vi "ECHGEI.vi"() -> ()   [LabVIEW 2018]
uses:
  S4GEI/S4GEI.lvclass
  S4GEI/S4GEI.lvclass/S4GEI.ctl
  Channel GUI/Channel.lvclass/Channel.ctl
  Channel GUI/Channel.lvclass
  Camera/Camera.lvclass
panel:
  in  "Tab Control 2":enum32{"Front Panel", "Setup Panel"}(tab)
  in  "Stop Application":bool
  out "Error Message":string
  in  "start exp":bool
  in  "Stop Acquisition":bool
  in  "Abort Acquisition":bool
  in  "Pause acquisition":bool
  in  "exp time":dbl=1.5 min=9.999999747378752e-06
  in  "#frames":u16=1 min=1 max=1000
  in  "#cycles":u32=1 min=1
  in  "Send Message":bool
  in  "Command:":string
  in  "ACS IP":string="200.131.64.25"
  in  "Channel ID":u16=1 min=1
  out "CCD status":T1={"Cycles done"=1, "Frames done"=1, "CCD Status"="", "Exposing"=FALSE, "Last image"="", "temp"=0, "serial n"=0, "texp"=0.0, "used disk"=0, "power"=FALSE, "acs mode"=FALSE} {"Frames done" max=2 scale=0.0..1.0; "Cycles done" max=2 scale=0.0..1.0}
  in  "projid":string="ENG"
  in  "observer":string="Denis"
  in  "object name":string="Test"
  in  "comment":string
  in  "file name suffix":string
  in  "preset modes":T2
  in  "Cooler":bool
  in  "Temp":i32=20 min=-80 max=20
  in  "Set camera configuration":bool
  in  "Readout Rate":u8(ring) items=["1 MHz", "0.1 MHz"]
  in  "Pre-amp gain":u8(ring) items=["Gain 1", "Gain 2", "Error"]
  in  "Vertical Clock Voltagem":u16(ring) items=["Normal", "+1", "+2", "+3", "+4", "Error"]
  in  "Acquisition Mode":u16(ring)=3 items=["Reserved", "Single Scan", "Accumulate", "Kinetic", "Fast Kinetic", "Run till abort", "Reserved", "Reserved", "Reserved", "Time Delayed Integration"]
  in  "Read Mode":u16(ring)=4 items=["Full Vertical Binning", "Multi-Track", "Random-Track", "Single-Track", "Image"]
  in  "Trigger Mode":u16(ring) items=["Internal", "External", "N/A", "N/A", "N/A", "N/A", "External Start", "External Exposure (Bulb)", "N/A", "External FVB EM", "Software", "N/A", "External Charge Shifting"]
  in  "Vertical Shift Speed":u16(ring)=3 items=["0.6", "1.13", "2.2", "4.33", "Error"]
  in  "AD Channel":u16
  in  "Shutter Mode":u8(ring)=2 items=["OPEN"=1, "CLOSED"=2, "Error"=3]
  in  "Shutter Time":u16=50
  in  "Shutter TTL":u16(ring) items=["TTL Low", "TTL High", "Error"]
  in  "Binning":u16=1
  in  "Initial Line":u16=1
  in  "Initial Cloumn":u16=1
  in  "Final Column":u16=1024
  in  "Final Line":u16=1024
  in  "Sub Image":T3(radio)=enum."1024 x 1024"
  # "ECHARPE Graphical Engineering Interface (ECHGEI)"
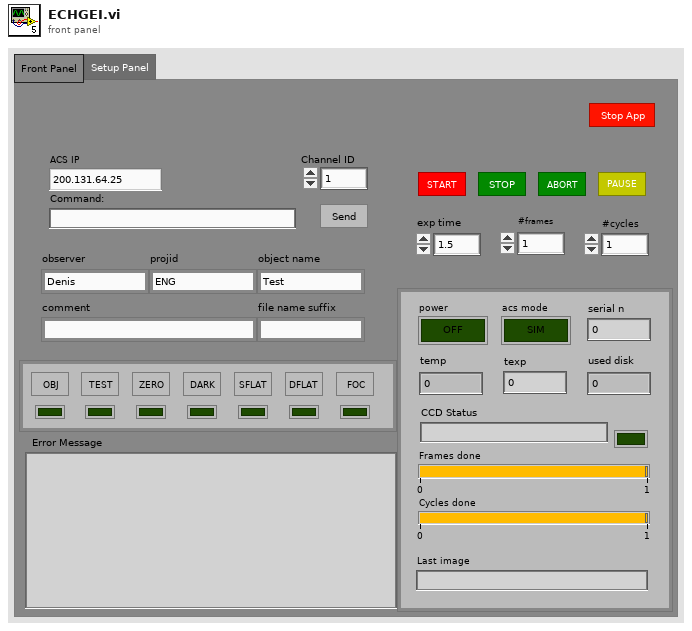
[diagram p1: front panel]
types:
  T1 = cluster{"Cycles done":u16, "Frames done":u16, "CCD Status":string, "Exposing":bool, "Last image":string, "temp":i16, "serial n":u16, "texp":dbl, "used disk":i16, "power":bool, "acs mode":bool}
  T2 = cluster{"OBJECT":bool, "TEST":bool, "ZERO":bool, "DARK":bool, "SFLAT":bool, "DFLAT":bool, "FOCUS":bool, "led object":bool, "led test":bool, "led zero":bool, "led dark":bool, "led sflat":bool, "led dflat":bool, "led foc":bool}
  T3 = enum32{"256 x 256", "512 x 512", "1024 x 1024", "Custom"}
  T4 = cluster{"FWCS IP":string, "ACS IP":string, "Channel ID":u16}
  T5 = cluster{"object":bool, "test":bool, "zero":bool, "dark":bool, "sflat":bool, "dflat":bool, "focus":bool, "object 2":bool, "test 2":bool, "zero 2":bool, "dark 2":bool, "sflat 2":bool, "dflat 2":bool, "foc":bool}
  T6 = enum8{"Enabled", "Disabled", "Disabled and Grayed Out"}
  T7 = cluster{"OBJECT":bool, "TEST":bool, "ZERO":bool, "DARK":bool, "SFLAT":bool, "DFLAT":bool, "FOCUS":bool}
  T8 = cluster{"CYCLES_DONE":u16, "LAST_IMAGE_NAME":string, "USED_DISK_SPACE":u16, "FRAMES_DONE":u16, "CCD_STATUS":string, "CURRENT_TEMPERATURE":i16, "TEMPERATURE_STATUS":string, "FRAME_EXPOSURE_TIME":sgl, "ERROR":bool, "SERIAL_NUMBER":u16, "ACQUIRING":bool, "IMAGE_INDEX":u32, "POWER":bool, "ACS MODE":bool}
  T9 = cluster{"PREAMP":u16, "READOUT_RATE":u16, "VERTICAL_SHIFT_SPEED":u16, "READ_MODE":u16, "VERTICAL_CLOCK_VOLTAGE":u16, "ACQUISITION_MODE":u16, "AD_CHANNEL":u16, "SHUTTER_TTL":u16, "SHUTTER_OPENING_TIME":u16, "SHUTTER_CLOSING_TIME":u16, "SHUTTER_MODE":u16, "TRIGGER_MODE":u16, "VBIN":u16, "INITIAL_LINE":u16, "INITIAL_COLUMN":u16, "FINAL_LINE":u16, "FINAL_COLUMN":u16, "HBIN":u16}
  T10 = cluster{"EXPTIME":dbl, "#FRAMES":u32, "#CYCLES":u32, "suffix":string, "TEMP":i32, "COOLER_POWER_STATUS":u16}
  T11 = cluster{"Acquire":bool, "Stop Acquisition":bool, "Abort Acquisition":bool, "Pause acquisition":bool}
  T12 = cluster{"OBJECT":string, "OBSERVER":string, "CTRLINTE":string, "PROJID":string, "SYNCMODE":string, "INSTMODE":string, "FILTER":string, "OBSTYPE":string, "GUIVRSN":string, "COMMENT":string, "broker":string, "timestamp":string, "CHANNEL 1":bool, "CHANNEL 2":bool, "CHANNEL 3":bool, "CHANNEL 4":bool, "TCSMODE":bool}
  T13 = cluster{"Cycles done":u16, "Frames done":u16, "CCD Status":string, "Exposing":bool, "Last image":string, "temp":i16, "serial n":u16, "texp":dbl, "used disk":i16, "Power":bool, "ACS mode":bool}
  T14 = cluster{"object":bool, "test":bool, "zero":bool, "dark":bool, "sflat":bool, "dflat":bool, "focus":bool, "led object":bool, "led test":bool, "led zero":bool, "led dark":bool, "led sflat":bool, "led dflat":bool, "led foc":bool}
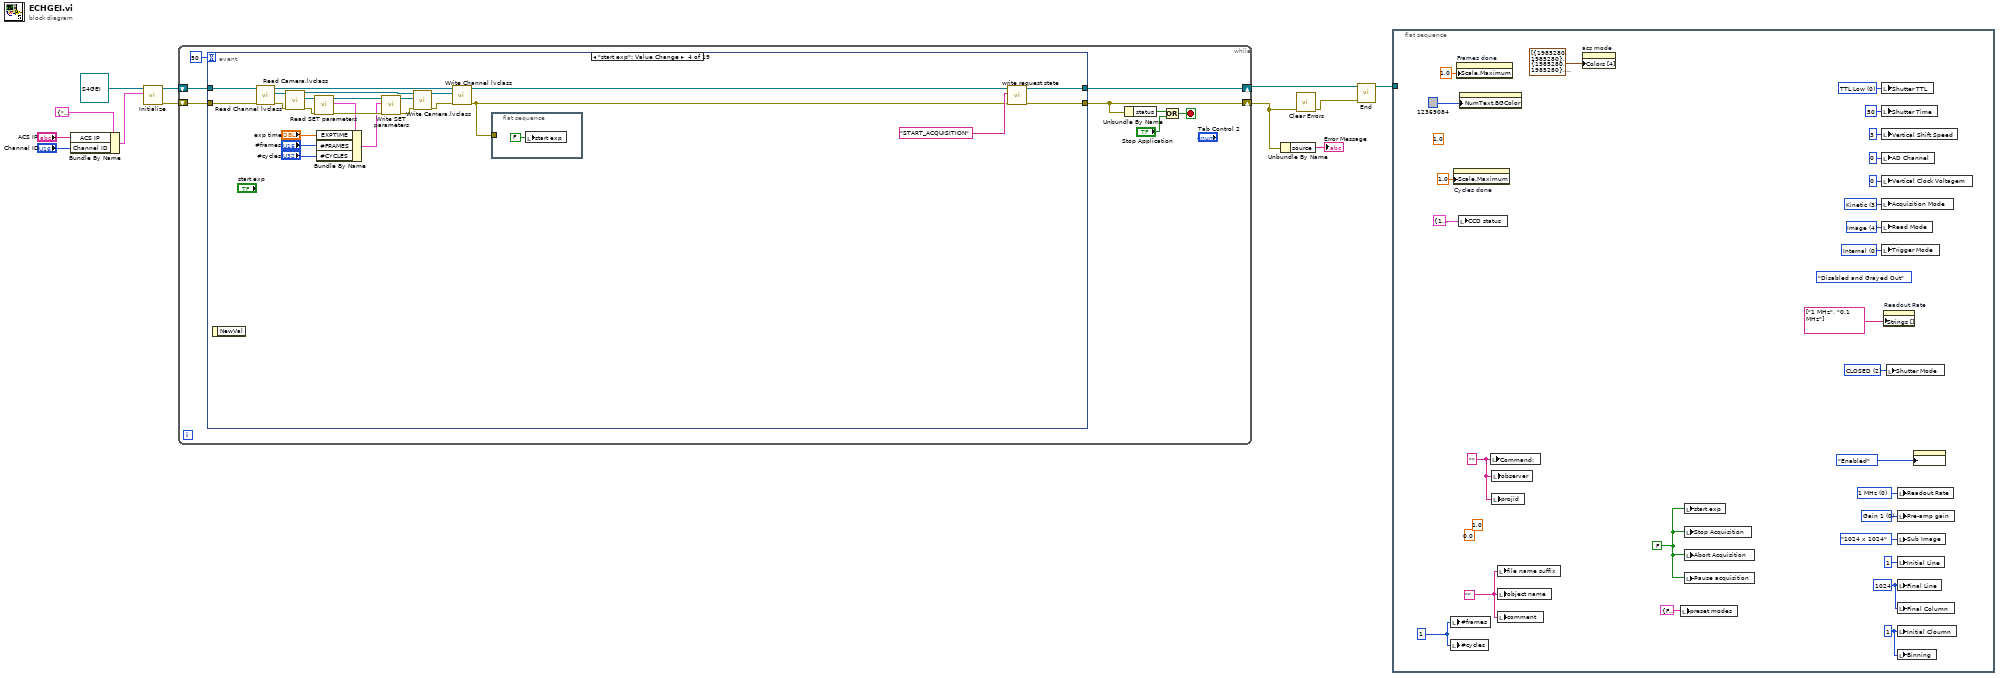
[diagram p0: block diagram]
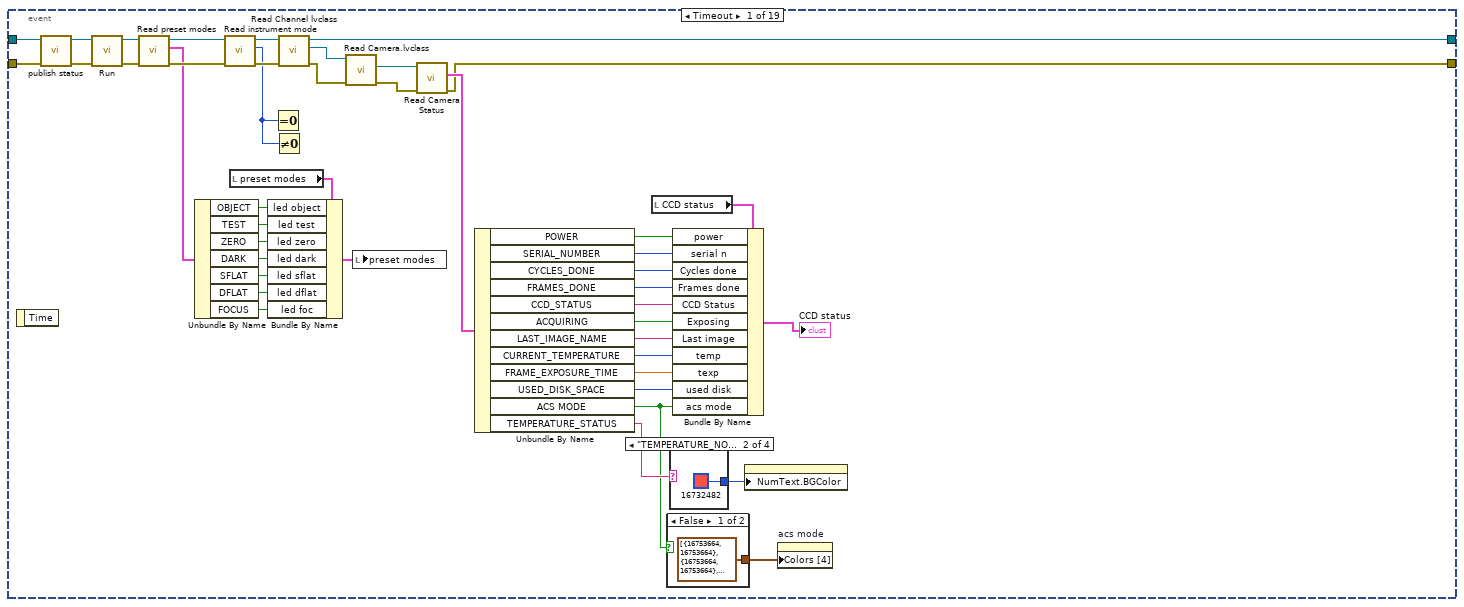
[diagram p2: hidden frame]
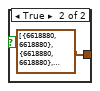
[diagram p3: hidden frame]
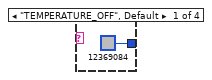
[diagram p4: hidden frame]
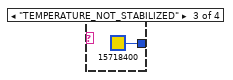
[diagram p5: hidden frame]
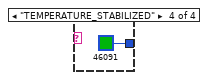
[diagram p6: hidden frame]
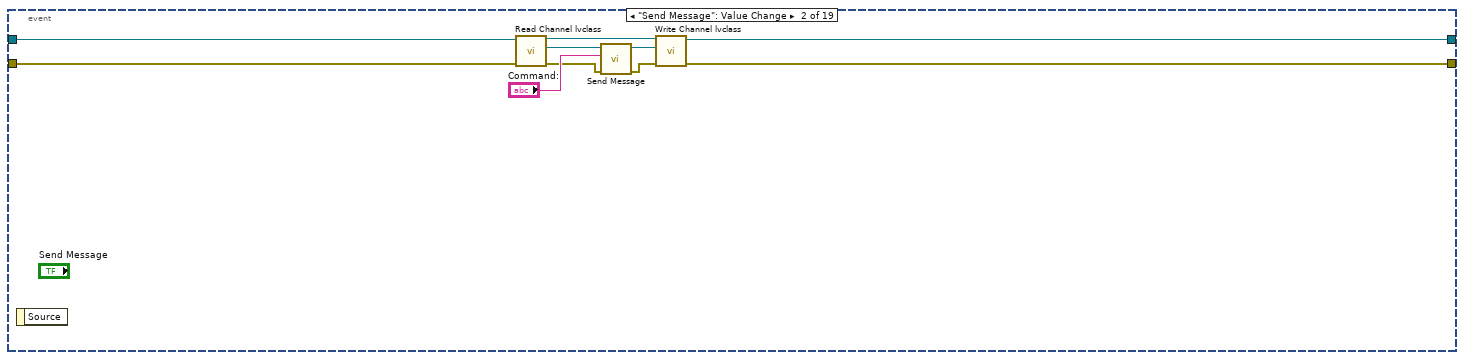
[diagram p7: hidden frame]
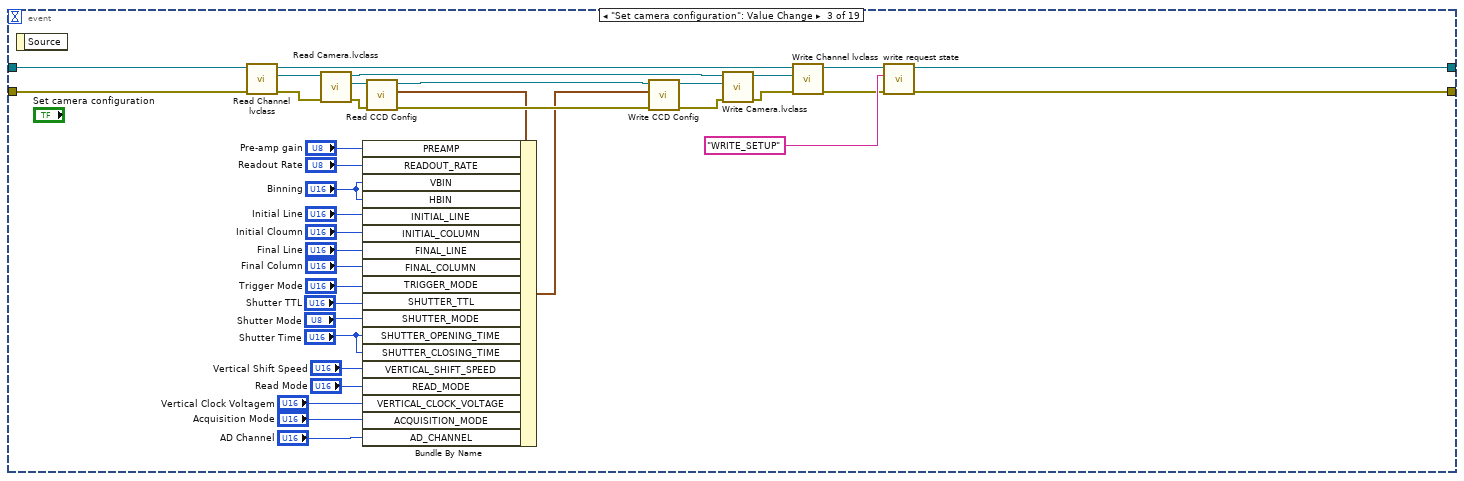
[diagram p8: hidden frame]
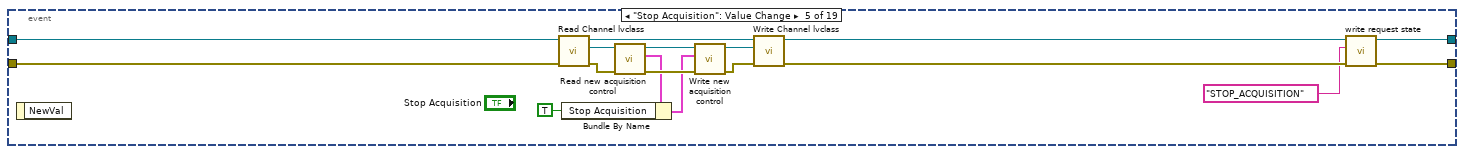
[diagram p9: hidden frame]
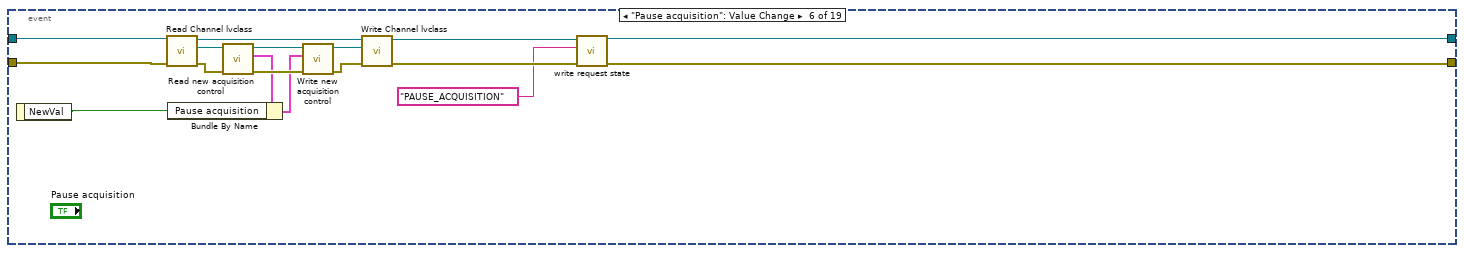
[diagram p10: hidden frame]
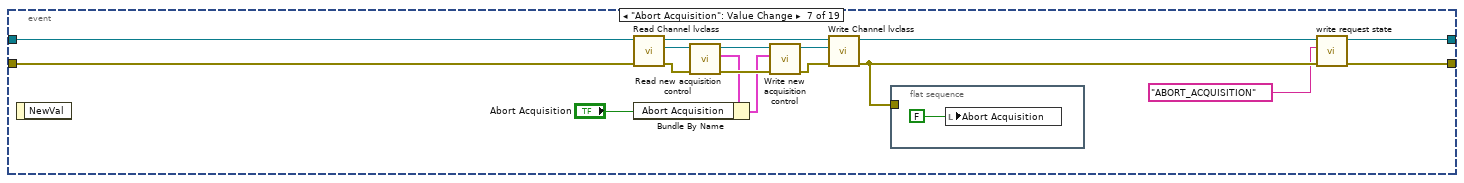
[diagram p11: hidden frame]
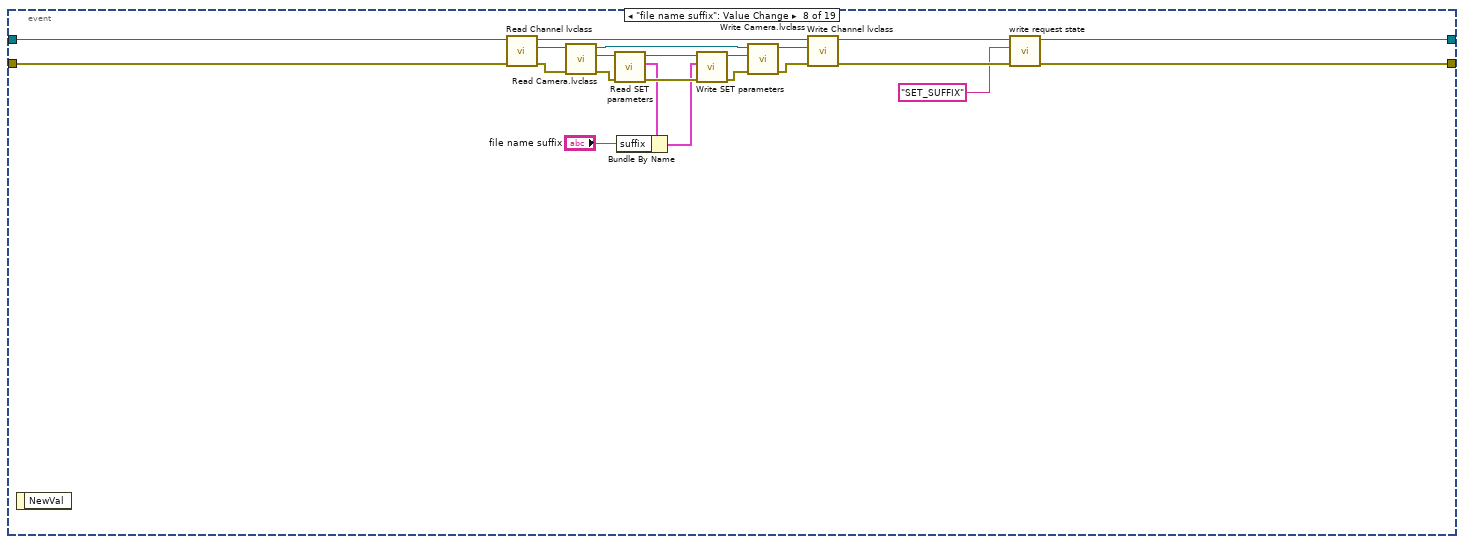
[diagram p12: hidden frame]
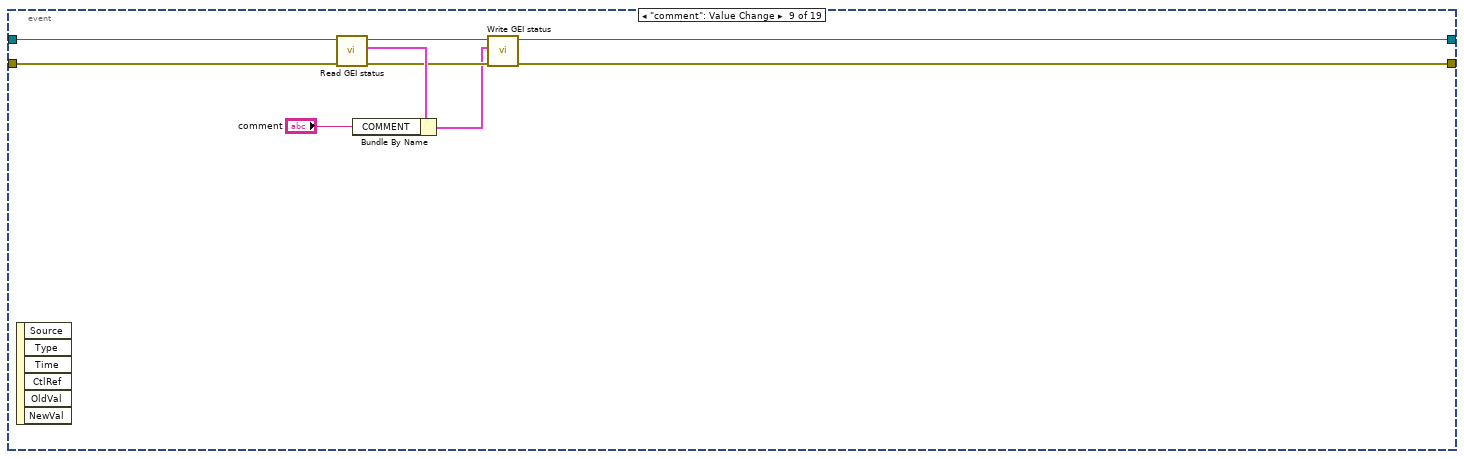
[diagram p13: hidden frame]
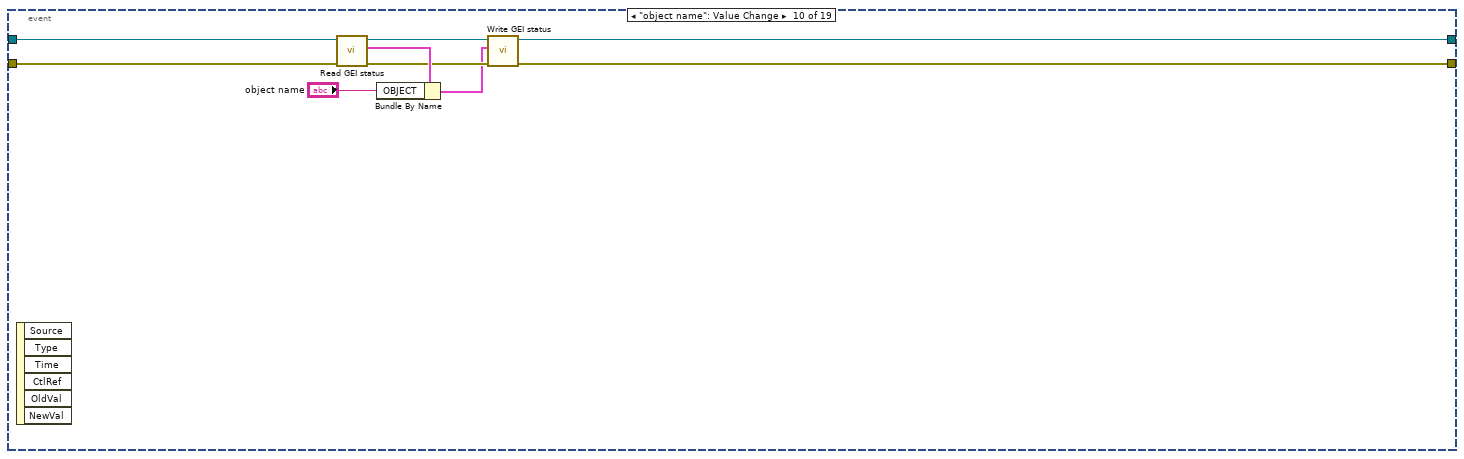
[diagram p14: hidden frame]
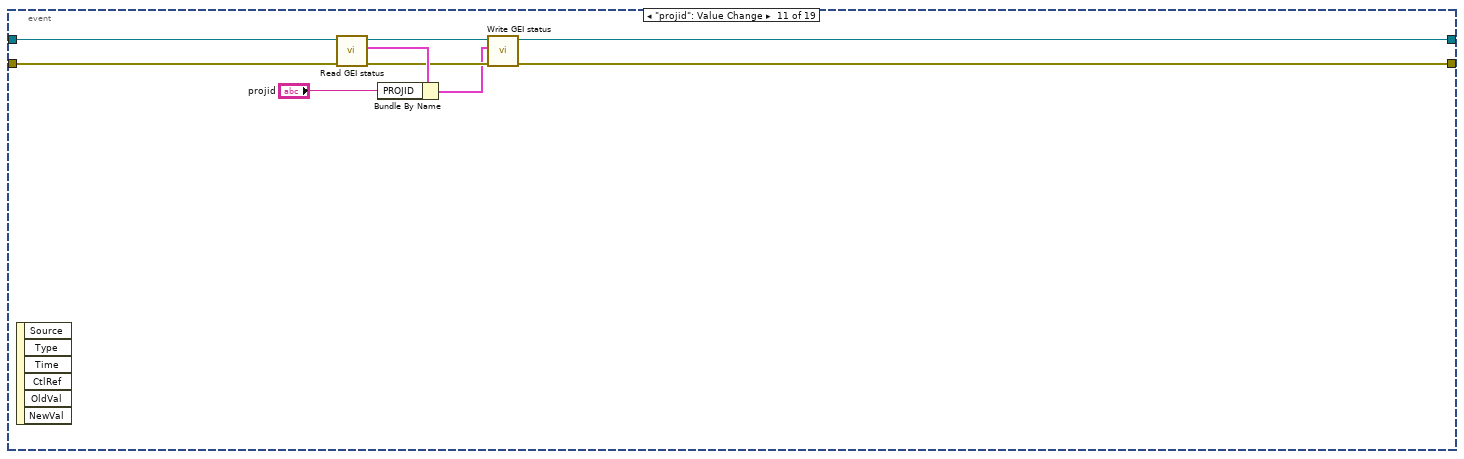
[diagram p15: hidden frame]
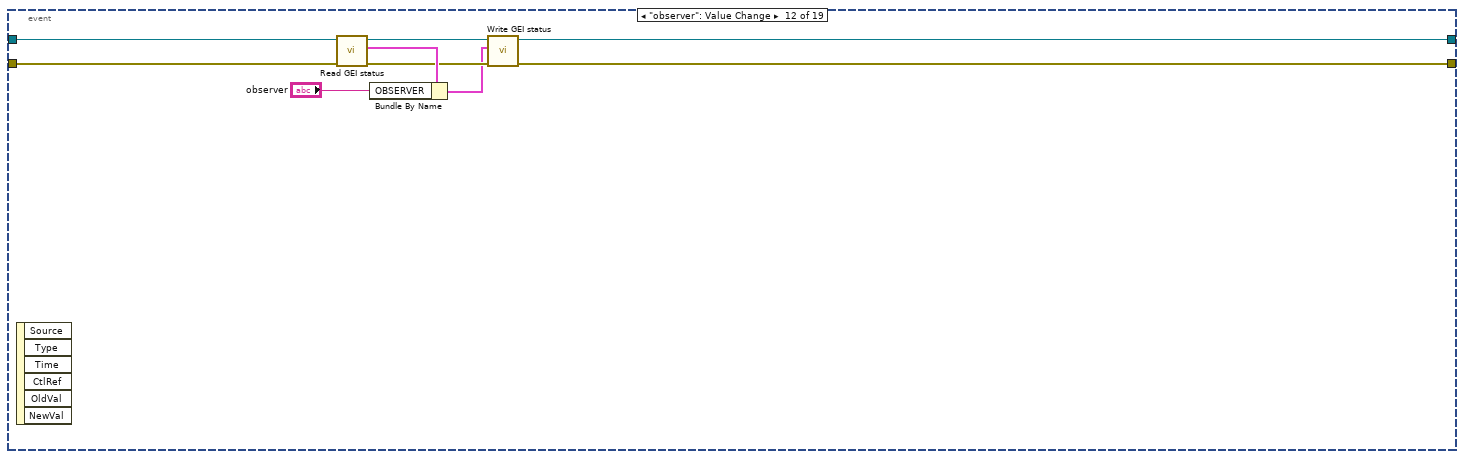
[diagram p16: hidden frame]
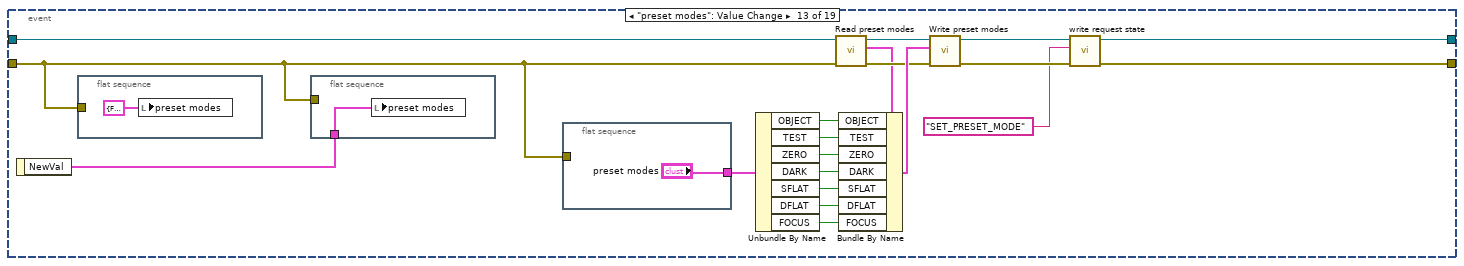
[diagram p17: hidden frame]
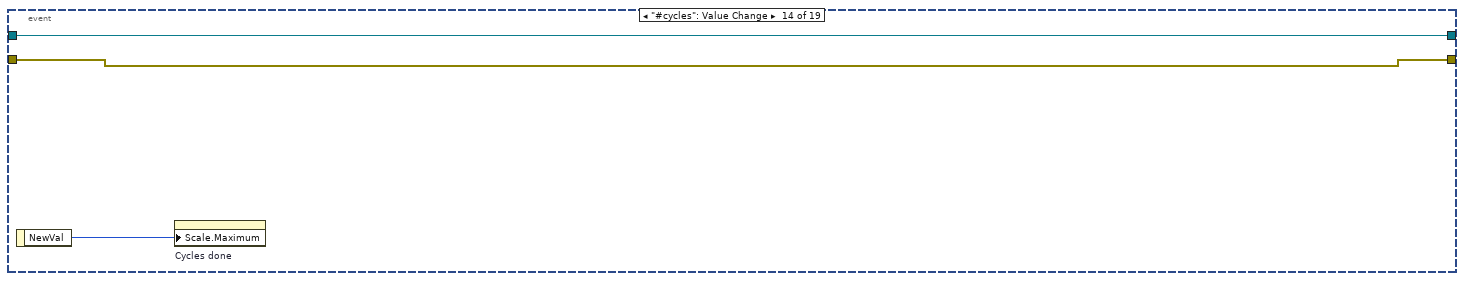
[diagram p18: hidden frame]
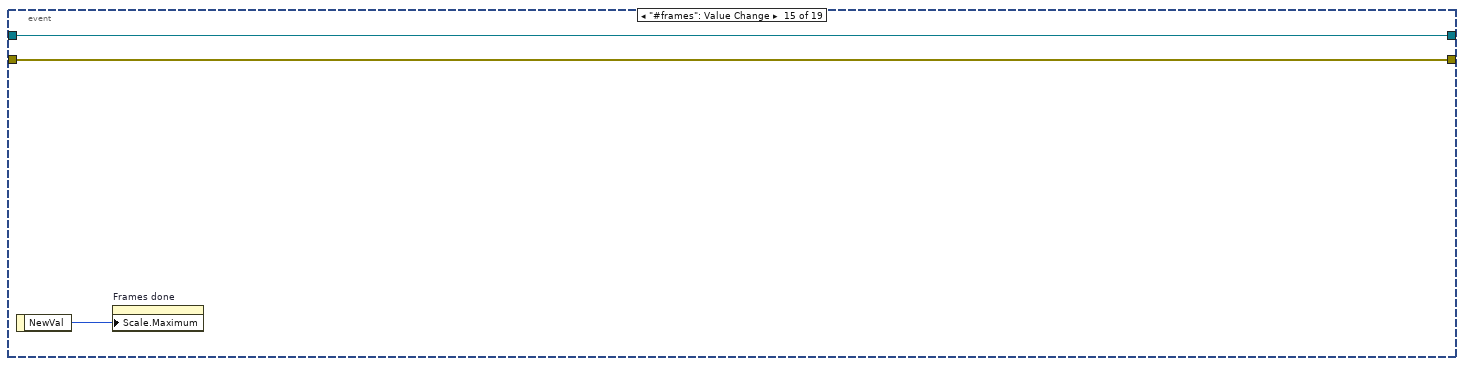
[diagram p19: hidden frame]
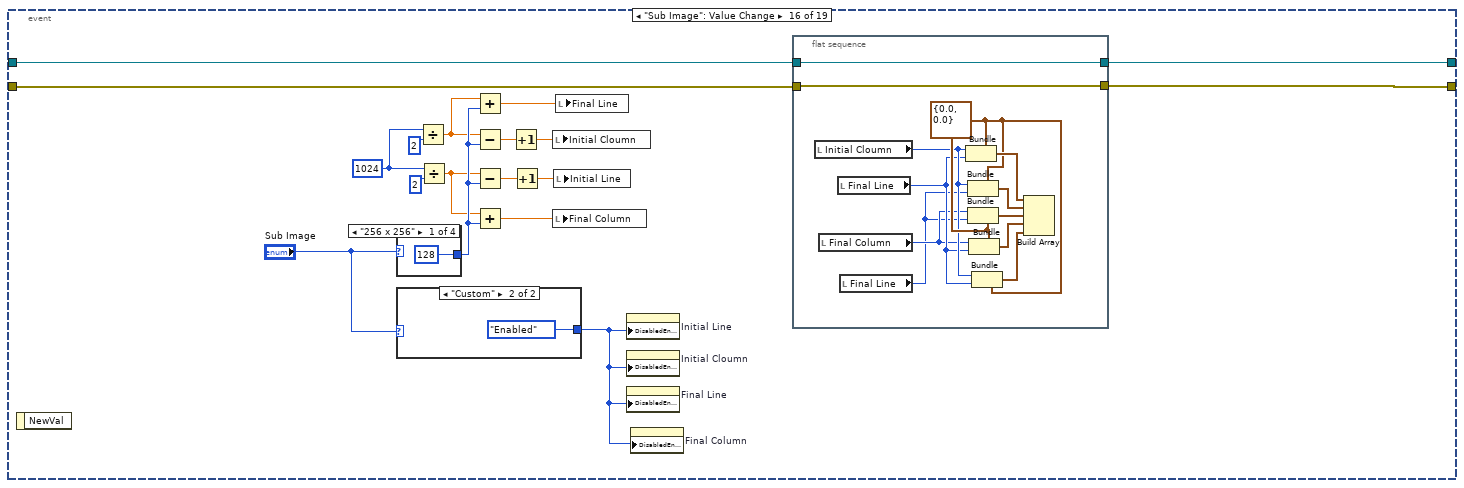
[diagram p20: hidden frame]
diagram:
  n1 = Bundle By Name(cluster=T4 {"FWCS IP"="200.131.64.49", "ACS IP"="200.131.64.25", "Channel ID"=1} ("Communication variables"), "ACS IP"="ACS IP", "Channel ID"="Channel ID") -> (w6:T4)
  n2 = call "Initialize.vi"("Communication variables"=w6, "SPARC4_GUI in"=refnum<class "S4GEI.lvclass"> refnum ("SPARC4_GUI.lvclass")) -> ("error out"=w2:errorcluster, "SPARC4_GUI out"=w1:refnum<class "S4GEI.lvclass">)  [unwired: 8 in]
  n3 = while {
    shift-right: [w13] -> w9
    shift-left: w2 -> [w15]
    shift-right: [w14] -> w11
    shift-left: w1 -> [w16]
    stop <- w19 stop-if-true
    n4 = event shown="[3] \"start exp\": Value Change" {
      selector: _ -> [_ _ _ _ _ _ _ _ _ _ _ _ _ _ _ _ _ _ _]
      dyn-events: _ -> [_ _ _ _ _ _ _ _ _ _ _ _ _ _ _ _ _ _ _]
      timeout: 50 -> [_ _ _ _ _ _ _ _ _ _ _ _ _ _ _ _ _ _ _]
      tunnel: w15 -> [w61 w78 w116 w139 w157 w166 w183 w215 w222 w231 w240 w249 w262 w277 w280 w298 w321 w339 w361]
      tunnel: [w40 w71 w82 w124 w147 w162 w178 w196 w223 w232 w241 w250 w269 w277 w280 w296 w321 w325 w349] -> w13
      tunnel: w16 -> [w62 w79 w117 w140 w158 w167 w184 w214 w224 w233 w242 w251 w261 w278 w281 w299 w320 w340 w362]
      tunnel: [w44 w72 w81 w125 w148 w161 w179 w197 w225 w234 w243 w252 w268 w278 w281 w297 w320 w326 w350] -> w14
      event Timeout {
        n5 = event-data() -> ()  [unwired: 1 in, 1 out]
        n6 = call "publish status.vi"("error in (no error)"=w61, "S4GEI in"=w62) -> ("error out"=w60:errorcluster, "S4GEI out"=w59:refnum<class "S4GEI.lvclass">)  [unwired: 8 in]
        n7 = call "Run.vi"("error in (no error)"=w60, "SPARC4_GUI in"=w59) -> ("error out"=w36:errorcluster, "SPARC4_GUI out"=w39:refnum<class "S4GEI.lvclass">)  [unwired: 8 in]
        n8 = call-dynamic "Read preset modes.vi"("error in (no error)"=w36, "S4GEI in"=w39) -> ("error out"=w37:errorcluster, "preset modes"=w33:T7, "S4GEI out"=w38:refnum<class "S4GEI.lvclass">)  [unwired: 7 in]
        n9 = Unbundle By Name(w33) -> ("OBJECT"=w26:bool, "TEST"=w27:bool, "ZERO"=w28:bool, "DARK"=w29:bool, "SFLAT"=w30:bool, "DFLAT"=w31:bool, "FOCUS"=w32:bool)
        n10 = call-dynamic "Read instrument mode.vi"("error in (no error)"=w37, "S4GEI in"=w38) -> ("error out"=w42:errorcluster, "instrument mode"=w41:u16, "S4GEI out"=w43:refnum<class "S4GEI.lvclass">)  [unwired: 7 in]
        n11 = local read "preset modes"() -> (w35:T2)
        n12 = Bundle By Name(cluster=w35, "led object"=w26, "led test"=w27, "led zero"=w28, "led dark"=w29, "led sflat"=w30, "led dflat"=w31, "led foc"=w32) -> (w34:T2)
        n13 = Equal To 0?(x=w41) -> ()  [unwired: 1 out]
        n14 = Not Equal To 0?(x=w41) -> ()  [unwired: 1 out]
        n15 = call "Read Channel lvclass.vi"("error in (no error)"=w42, "SPARC4_GUI in"=w43) -> ("error out"=w56:errorcluster, "Channel.lvclass"=w58:refnum<class "Channel.lvclass">, "SPARC4_GUI out"=w44:refnum<class "S4GEI.lvclass">)  [unwired: 7 in]
        n16 = call-dynamic "Read Camera.lvclass.vi"("error in (no error)"=w56, "Channel in"=w58) -> ("error out"=w55:errorcluster, "Camera.lvclass"=w57:refnum<class "Camera.lvclass">)  [unwired: 7 in, 1 out]
        n17 = local write "preset modes"(w34) -> ()
        n18 = call-dynamic "Read Camera Status.vi"("error in (no error)"=w55, "Camera in"=w57) -> ("error out"=w40:errorcluster, "Camera Status"=w63:T8)  [unwired: 7 in, 1 out]
        n19 = Unbundle By Name(w63) -> ("POWER"=w24:bool, "SERIAL_NUMBER"=w25:u16, "CYCLES_DONE"=w52:u16, "FRAMES_DONE"=w51:u16, "CCD_STATUS"=w50:string, "ACQUIRING"=w49:bool, "LAST_IMAGE_NAME"=w48:string, "CURRENT_TEMPERATURE"=w47:i16, "FRAME_EXPOSURE_TIME"=w46:sgl, "USED_DISK_SPACE"=w45:u16, "ACS MODE"=w21:bool, "TEMPERATURE_STATUS"=w23:string)
        n20 = local read "CCD status"() -> (w54:T1)
        n21 = case shown="False" w21 {
          tunnel: [cluster{u32, u32}[] [{16753664, 16753664}, {16753664, 16753664}, {16753664, 16753664}] ("Colors [4]") cluster{u32, u32}[] [{6618880, 6618880}, {6618880, 6618880}, {6618880, 6618880}] ("Colors [4]")] -> w22
          frame False {
          }
          frame True {
          }
        }
        n22 = case shown="\"TEMPERATURE_NOT_REACHED\"" w23 {
          tunnel: [u32 12369084 u32 16732482 u32 15718400 u32 46091] -> w64
          frame "TEMPERATURE_OFF", Default {
          }
          frame "TEMPERATURE_NOT_REACHED" {
          }
          frame "TEMPERATURE_NOT_STABILIZED" {
          }
          frame "TEMPERATURE_STABILIZED" {
          }
        }
        n23 = Bundle By Name(cluster=w54, "power"=w24, "serial n"=w25, "Cycles done"=w52, "Frames done"=w51, "CCD Status"=w50, "Exposing"=w49, "Last image"=w48, "temp"=w47, "texp"=w46, "used disk"=w45, "acs mode"=w21) -> (→"CCD status":T1)
        n24 = property on="temp" class="DigNum (strict)"("NumText.BGColor"=w64) -> ()  [unwired: 2 in, 2 out]
        n25 = property on="acs mode" class="Bool (strict)"("Colors [4]"=w22) -> ()  [unwired: 2 in, 2 out]
      }
      event "Send Message": Value Change {
        n26 = event-data() -> ()  [unwired: 1 in, 1 out]
        n27 = call "Read Channel lvclass.vi"("error in (no error)"=w78, "SPARC4_GUI in"=w79) -> ("error out"=w74:errorcluster, "Channel.lvclass"=w77:refnum<class "Channel.lvclass">, "SPARC4_GUI out"=w73:refnum<class "S4GEI.lvclass">)  [unwired: 7 in]
        n28 = call "Send Message.vi"("error in (no error)"=w74, "Message"="Command:", "Channel GUI in"=w77) -> ("error out"=w75:errorcluster, "Channel GUI out"=w76:refnum<class "Channel.lvclass">)  [unwired: 7 in]
        n29 = call "Write Channel lvclass.vi"("error in (no error)"=w75, "Channel.lvclass"=w76, "SPARC4_GUI in"=w73) -> ("error out"=w71:errorcluster, "SPARC4_GUI out"=w72:refnum<class "S4GEI.lvclass">)  [unwired: 7 in]
      }
      event "Set camera configuration": Value Change {
        n30 = event-data() -> ()  [unwired: 1 in, 1 out]
        n31 = call "Read Channel lvclass.vi"("error in (no error)"=w116, "SPARC4_GUI in"=w117) -> ("error out"=w115:errorcluster, "Channel.lvclass"=w87:refnum<class "Channel.lvclass">, "SPARC4_GUI out"=w114:refnum<class "S4GEI.lvclass">)  [unwired: 7 in]
        n32 = call-dynamic "Read Camera.lvclass.vi"("error in (no error)"=w115, "Channel in"=w87) -> ("error out"=w113:errorcluster, "Camera.lvclass"=w112:refnum<class "Camera.lvclass">, "Channel out"=w86:refnum<class "Channel.lvclass">)  [unwired: 7 in]
        n33 = call-dynamic "Read CCD Config.vi"("error in (no error)"=w113, "Camera in"=w112) -> ("error out"=w111:errorcluster, "CCD Config"=w89:T9, "Camera out"=w94:refnum<class "Camera.lvclass">)  [unwired: 7 in]
        n34 = Bundle By Name(cluster=w89, "PREAMP"="Pre-amp gain", "READOUT_RATE"="Readout Rate", "VBIN"="Binning", "HBIN"="Binning", "INITIAL_LINE"="Initial Line", "INITIAL_COLUMN"="Initial Cloumn", "FINAL_LINE"="Final Line", "FINAL_COLUMN"="Final Column", "TRIGGER_MODE"="Trigger Mode", "SHUTTER_TTL"="Shutter TTL", "SHUTTER_MODE"="Shutter Mode", "SHUTTER_OPENING_TIME"="Shutter Time", "SHUTTER_CLOSING_TIME"="Shutter Time", "VERTICAL_SHIFT_SPEED"="Vertical Shift Speed", "READ_MODE"="Read Mode", "VERTICAL_CLOCK_VOLTAGE"="Vertical Clock Voltagem", "ACQUISITION_MODE"="Acquisition Mode", "AD_CHANNEL"="AD Channel") -> (w88:T9)
        n35 = call-dynamic "Write CCD Config.vi"("error in (no error)"=w111, "CCD Config"=w88, "Camera in"=w94) -> ("error out"=w92:errorcluster, "Camera out"=w93:refnum<class "Camera.lvclass">)  [unwired: 7 in]
        n36 = call-dynamic "Write Camera.lvclass.vi"("error in (no error)"=w92, "Camera.lvclass"=w93, "Channel in"=w86) -> ("error out"=w91:errorcluster, "Channel out"=w90:refnum<class "Channel.lvclass">)  [unwired: 7 in]
        n37 = call "Write Channel lvclass.vi"("error in (no error)"=w91, "Channel.lvclass"=w90, "SPARC4_GUI in"=w114) -> ("error out"=w84:errorcluster, "SPARC4_GUI out"=w83:refnum<class "S4GEI.lvclass">)  [unwired: 7 in]
        n38 = call "write request state.vi"("error in (no error)"=w84, "State"="WRITE_SETUP", "S4GEI in"=w83) -> ("error out"=w82:errorcluster, "S4GEI out"=w81:refnum<class "S4GEI.lvclass">)  [unwired: 7 in]
      }
      event "start exp": Value Change {
        n39 = event-data() -> ()  [unwired: 1 in, 1 out]
        n40 = call "Read Channel lvclass.vi"("error in (no error)"=w139, "SPARC4_GUI in"=w140) -> ("error out"=w138:errorcluster, "Channel.lvclass"=w127:refnum<class "Channel.lvclass">, "SPARC4_GUI out"=w141:refnum<class "S4GEI.lvclass">)  [unwired: 7 in]
        n41 = call-dynamic "Read Camera.lvclass.vi"("error in (no error)"=w138, "Channel in"=w127) -> ("error out"=w134:errorcluster, "Camera.lvclass"=w135:refnum<class "Camera.lvclass">, "Channel out"=w126:refnum<class "Channel.lvclass">)  [unwired: 7 in]
        n42 = call-dynamic "Read SET parameters.vi"("error in (no error)"=w134, "Camera in"=w135) -> ("error out"=w132:errorcluster, "SET parameters"=w129:T10, "Camera out"=w133:refnum<class "Camera.lvclass">)  [unwired: 7 in]
        n43 = Bundle By Name(cluster=w129, "EXPTIME"="exp time", "#FRAMES"="#frames", "#CYCLES"="#cycles") -> (w128:T10)
        n44 = call-dynamic "Write SET parameters.vi"("error in (no error)"=w132, "SET parameters"=w128, "Camera in"=w133) -> ("error out"=w130:errorcluster, "Camera out"=w131:refnum<class "Camera.lvclass">)  [unwired: 7 in]
        n45 = call-dynamic "Write Camera.lvclass.vi"("error in (no error)"=w130, "Camera.lvclass"=w131, "Channel in"=w126) -> ("error out"=w137:errorcluster, "Channel out"=w136:refnum<class "Channel.lvclass">)  [unwired: 7 in]
        n46 = call "Write Channel lvclass.vi"("error in (no error)"=w137, "Channel.lvclass"=w136, "SPARC4_GUI in"=w141) -> ("error out"=w121:errorcluster, "SPARC4_GUI out"=w122:refnum<class "S4GEI.lvclass">)  [unwired: 7 in]
        n47 = flat-sequence {
          tunnel: w121 -> [_]
          frame #0 {
            n48 = local write "start exp"(FALSE ("start exp")) -> ()
          }
        }
        n49 = call "write request state.vi"("error in (no error)"=w121, "State"="START_ACQUISITION", "S4GEI in"=w122) -> ("error out"=w124:errorcluster, "S4GEI out"=w125:refnum<class "S4GEI.lvclass">)  [unwired: 7 in]
      }
      event "Stop Acquisition": Value Change {
        n50 = event-data() -> ()  [unwired: 1 in, 1 out]
        n51 = call "Read Channel lvclass.vi"("error in (no error)"=w157, "SPARC4_GUI in"=w158) -> ("error out"=w153:errorcluster, "Channel.lvclass"=w156:refnum<class "Channel.lvclass">, "SPARC4_GUI out"=w159:refnum<class "S4GEI.lvclass">)  [unwired: 7 in]
        n52 = call "Read new acquisition control.vi"("error in (no error)"=w153, "Channel in"=w156) -> ("error out"=w152:errorcluster, "new acquisition control"=w150:T11, "Channel out"=w155:refnum<class "Channel.lvclass">)  [unwired: 7 in]
        n53 = Bundle By Name(cluster=w150, "Stop Acquisition"=TRUE) -> (w149:T11)
        n54 = call "Write new acquisition control.vi"("error in (no error)"=w152, "new acquisition control"=w149, "Channel in"=w155) -> ("error out"=w151:errorcluster, "Channel out"=w154:refnum<class "Channel.lvclass">)  [unwired: 7 in]
        n55 = call "Write Channel lvclass.vi"("error in (no error)"=w151, "Channel.lvclass"=w154, "SPARC4_GUI in"=w159) -> ("error out"=w146:errorcluster, "SPARC4_GUI out"=w145:refnum<class "S4GEI.lvclass">)  [unwired: 7 in]
        n56 = call "write request state.vi"("error in (no error)"=w146, "State"="STOP_ACQUISITION", "S4GEI in"=w145) -> ("error out"=w147:errorcluster, "S4GEI out"=w148:refnum<class "S4GEI.lvclass">)  [unwired: 7 in]
      }
      event "Pause acquisition": Value Change {
        n57 = event-data() -> ("NewVal"=w165:bool)  [unwired: 1 in]
        n58 = call "Read Channel lvclass.vi"("error in (no error)"=w166, "SPARC4_GUI in"=w167) -> ("error out"=w172:errorcluster, "Channel.lvclass"=w175:refnum<class "Channel.lvclass">, "SPARC4_GUI out"=w176:refnum<class "S4GEI.lvclass">)  [unwired: 7 in]
        n59 = call "Read new acquisition control.vi"("error in (no error)"=w172, "Channel in"=w175) -> ("error out"=w171:errorcluster, "new acquisition control"=w169:T11, "Channel out"=w174:refnum<class "Channel.lvclass">)  [unwired: 7 in]
        n60 = Bundle By Name(cluster=w169, "Pause acquisition"=w165) -> (w168:T11)
        n61 = call "Write new acquisition control.vi"("error in (no error)"=w171, "new acquisition control"=w168, "Channel in"=w174) -> ("error out"=w170:errorcluster, "Channel out"=w173:refnum<class "Channel.lvclass">)  [unwired: 7 in]
        n62 = call "Write Channel lvclass.vi"("error in (no error)"=w170, "Channel.lvclass"=w173, "SPARC4_GUI in"=w176) -> ("error out"=w164:errorcluster, "SPARC4_GUI out"=w163:refnum<class "S4GEI.lvclass">)  [unwired: 7 in]
        n63 = call "write request state.vi"("error in (no error)"=w164, "State"="PAUSE_ACQUISITION", "S4GEI in"=w163) -> ("error out"=w162:errorcluster, "S4GEI out"=w161:refnum<class "S4GEI.lvclass">)  [unwired: 7 in]
      }
      event "Abort Acquisition": Value Change {
        n64 = event-data() -> ()  [unwired: 1 in, 1 out]
        n65 = call "Read Channel lvclass.vi"("error in (no error)"=w183, "SPARC4_GUI in"=w184) -> ("error out"=w189:errorcluster, "Channel.lvclass"=w192:refnum<class "Channel.lvclass">, "SPARC4_GUI out"=w193:refnum<class "S4GEI.lvclass">)  [unwired: 7 in]
        n66 = call "Read new acquisition control.vi"("error in (no error)"=w189, "Channel in"=w192) -> ("error out"=w188:errorcluster, "new acquisition control"=w186:T11, "Channel out"=w191:refnum<class "Channel.lvclass">)  [unwired: 7 in]
        n67 = Bundle By Name(cluster=w186, "Abort Acquisition"="Abort Acquisition") -> (w185:T11)
        n68 = call "Write new acquisition control.vi"("error in (no error)"=w188, "new acquisition control"=w185, "Channel in"=w191) -> ("error out"=w187:errorcluster, "Channel out"=w190:refnum<class "Channel.lvclass">)  [unwired: 7 in]
        n69 = call "Write Channel lvclass.vi"("error in (no error)"=w187, "Channel.lvclass"=w190, "SPARC4_GUI in"=w193) -> ("error out"=w180:errorcluster, "SPARC4_GUI out"=w181:refnum<class "S4GEI.lvclass">)  [unwired: 7 in]
        n70 = flat-sequence {
          tunnel: w180 -> [_]
          frame #0 {
            n71 = local write "Abort Acquisition"(FALSE ("Abort Acquisition")) -> ()
          }
        }
        n72 = call "write request state.vi"("error in (no error)"=w180, "State"="ABORT_ACQUISITION", "S4GEI in"=w181) -> ("error out"=w178:errorcluster, "S4GEI out"=w179:refnum<class "S4GEI.lvclass">)  [unwired: 7 in]
      }
      event "file name suffix": Value Change {
        n73 = event-data() -> ()  [unwired: 1 in, 1 out]
        n74 = call "Read Channel lvclass.vi"("error in (no error)"=w215, "SPARC4_GUI in"=w214) -> ("error out"=w213:errorcluster, "Channel.lvclass"=w204:refnum<class "Channel.lvclass">, "SPARC4_GUI out"=w216:refnum<class "S4GEI.lvclass">)  [unwired: 7 in]
        n75 = call-dynamic "Read Camera.lvclass.vi"("error in (no error)"=w213, "Channel in"=w204) -> ("error out"=w209:errorcluster, "Camera.lvclass"=w210:refnum<class "Camera.lvclass">, "Channel out"=w203:refnum<class "Channel.lvclass">)  [unwired: 7 in]
        n76 = call-dynamic "Read SET parameters.vi"("error in (no error)"=w209, "Camera in"=w210) -> ("error out"=w208:errorcluster, "SET parameters"=w202:T10, "Camera out"=w207:refnum<class "Camera.lvclass">)  [unwired: 7 in]
        n77 = Bundle By Name(cluster=w202, "suffix"="file name suffix") -> (w201:T10)
        n78 = call-dynamic "Write SET parameters.vi"("error in (no error)"=w208, "SET parameters"=w201, "Camera in"=w207) -> ("error out"=w211:errorcluster, "Camera out"=w212:refnum<class "Camera.lvclass">)  [unwired: 7 in]
        n79 = call-dynamic "Write Camera.lvclass.vi"("error in (no error)"=w211, "Camera.lvclass"=w212, "Channel in"=w203) -> ("error out"=w205:errorcluster, "Channel out"=w206:refnum<class "Channel.lvclass">)  [unwired: 7 in]
        n80 = call "Write Channel lvclass.vi"("error in (no error)"=w205, "Channel.lvclass"=w206, "SPARC4_GUI in"=w216) -> ("error out"=w198:errorcluster, "SPARC4_GUI out"=w199:refnum<class "S4GEI.lvclass">)  [unwired: 7 in]
        n81 = call "write request state.vi"("error in (no error)"=w198, "State"="SET_SUFFIX" ("Message"), "S4GEI in"=w199) -> ("error out"=w196:errorcluster, "S4GEI out"=w197:refnum<class "S4GEI.lvclass">)  [unwired: 7 in]
      }
      event "comment": Value Change {
        n82 = event-data() -> ()  [unwired: 1 in, 6 out]
        n83 = call-dynamic "Read GEI status.vi"("error in (no error)"=w222, "S4GEI in"=w224) -> ("error out"=w220:errorcluster, "GEI status"=w221:T12, "S4GEI out"=w219:refnum<class "S4GEI.lvclass">)  [unwired: 7 in]
        n84 = Bundle By Name(cluster=w221, "COMMENT"="comment") -> (w218:T12)
        n85 = call-dynamic "Write GEI status.vi"("error in (no error)"=w220, "GEI status"=w218, "S4GEI in"=w219) -> ("error out"=w223:errorcluster, "S4GEI out"=w225:refnum<class "S4GEI.lvclass">)  [unwired: 7 in]
      }
      event "object name": Value Change {
        n86 = event-data() -> ()  [unwired: 1 in, 6 out]
        n87 = call-dynamic "Read GEI status.vi"("error in (no error)"=w231, "S4GEI in"=w233) -> ("error out"=w229:errorcluster, "GEI status"=w230:T12, "S4GEI out"=w228:refnum<class "S4GEI.lvclass">)  [unwired: 7 in]
        n88 = Bundle By Name(cluster=w230, "OBJECT"="object name") -> (w227:T12)
        n89 = call-dynamic "Write GEI status.vi"("error in (no error)"=w229, "GEI status"=w227, "S4GEI in"=w228) -> ("error out"=w232:errorcluster, "S4GEI out"=w234:refnum<class "S4GEI.lvclass">)  [unwired: 7 in]
      }
      event "projid": Value Change {
        n90 = event-data() -> ()  [unwired: 1 in, 6 out]
        n91 = call-dynamic "Read GEI status.vi"("error in (no error)"=w240, "S4GEI in"=w242) -> ("error out"=w238:errorcluster, "GEI status"=w239:T12, "S4GEI out"=w237:refnum<class "S4GEI.lvclass">)  [unwired: 7 in]
        n92 = Bundle By Name(cluster=w239, "PROJID"="projid") -> (w236:T12)
        n93 = call-dynamic "Write GEI status.vi"("error in (no error)"=w238, "GEI status"=w236, "S4GEI in"=w237) -> ("error out"=w241:errorcluster, "S4GEI out"=w243:refnum<class "S4GEI.lvclass">)  [unwired: 7 in]
      }
      event "observer": Value Change {
        n94 = event-data() -> ()  [unwired: 1 in, 6 out]
        n95 = call-dynamic "Read GEI status.vi"("error in (no error)"=w249, "S4GEI in"=w251) -> ("error out"=w247:errorcluster, "GEI status"=w248:T12, "S4GEI out"=w246:refnum<class "S4GEI.lvclass">)  [unwired: 7 in]
        n96 = Bundle By Name(cluster=w248, "OBSERVER"="observer") -> (w245:T12)
        n97 = call-dynamic "Write GEI status.vi"("error in (no error)"=w247, "GEI status"=w245, "S4GEI in"=w246) -> ("error out"=w250:errorcluster, "S4GEI out"=w252:refnum<class "S4GEI.lvclass">)  [unwired: 7 in]
      }
      event "preset modes": Value Change {
        n98 = event-data() -> ("NewVal"=w272:T2)  [unwired: 1 in]
        n99 = flat-sequence {
          tunnel: w262 -> [_]
          frame #0 {
            n100 = local write "preset modes"(T5 {"object"=FALSE, "test"=FALSE, "zero"=FALSE, "dark"=FALSE, "sflat"=FALSE, "dflat"=FALSE, "focus"=FALSE, "object 2"=FALSE, "test 2"=FALSE, "zero 2"=FALSE, "dark 2"=FALSE, "sflat 2"=FALSE, "dflat 2"=FALSE, "foc"=FALSE} ("preset modes")) -> ()
          }
        }
        n101 = flat-sequence {
          tunnel: w262 -> [_]
          tunnel: w272 -> [w274]
          frame #0 {
            n102 = local write "preset modes"(w274) -> ()
          }
        }
        n103 = flat-sequence {
          tunnel: w262 -> [_]
          tunnel: ["preset modes"] -> w260
          frame #0 {
          }
        }
        n104 = Unbundle By Name(w260) -> ("OBJECT"=w259:bool, "TEST"=w258:bool, "ZERO"=w257:bool, "DARK"=w256:bool, "SFLAT"=w255:bool, "DFLAT"=w254:bool, "FOCUS"=w253:bool)
        n105 = call-dynamic "Read preset modes.vi"("error in (no error)"=w262, "S4GEI in"=w261) -> ("error out"=w264:errorcluster, "preset modes"=w263:T7, "S4GEI out"=w265:refnum<class "S4GEI.lvclass">)  [unwired: 7 in]
        n106 = Bundle By Name(cluster=w263, "OBJECT"=w259, "TEST"=w258, "ZERO"=w257, "DARK"=w256, "SFLAT"=w255, "DFLAT"=w254, "FOCUS"=w253) -> (w266:T7)
        n107 = call-dynamic "Write preset modes.vi"("error in (no error)"=w264, "preset modes"=w266, "S4GEI in"=w265) -> ("error out"=w270:errorcluster, "S4GEI out"=w271:refnum<class "S4GEI.lvclass">)  [unwired: 7 in]
        n108 = call "write request state.vi"("error in (no error)"=w270, "State"="SET_PRESET_MODE", "S4GEI in"=w271) -> ("error out"=w269:errorcluster, "S4GEI out"=w268:refnum<class "S4GEI.lvclass">)  [unwired: 7 in]
      }
      event "#cycles": Value Change {
        n109 = event-data() -> ("NewVal"=w276:u32)  [unwired: 1 in]
        n110 = property on="Cycles done" class="Slide (strict)"("Scale.Maximum"=w276) -> ()  [unwired: 2 in, 2 out]
      }
      event "#frames": Value Change {
        n111 = event-data() -> ("NewVal"=w279:u16)  [unwired: 1 in]
        n112 = property on="Frames done" class="Slide (strict)"("Scale.Maximum"=w279) -> ()  [unwired: 2 in, 2 out]
      }
      event "Sub Image": Value Change {
        w286 = 1024
        n113 = event-data() -> ()  [unwired: 1 in, 1 out]
        n114 = case shown="\"256 x 256\"" "Sub Image" {
          tunnel: [128 256 512 512] -> w290
          frame "256 x 256" {
          }
          frame "512 x 512" {
          }
          frame "1024 x 1024", Default {
          }
          frame "Custom" {
          }
        }
        n115 = case shown="\"Custom\"" "Sub Image" {
          tunnel: [T6."Disabled and Grayed Out" ("Disabled") T6."Enabled" ("Disabled")] -> w293
          frame "1024 x 1024", Default {
          }
          frame "Custom" {
          }
        }
        n116 = Divide(x=w286, y=2) -> (x/y=w289:dbl)
        n117 = Divide(x=w286, y=2) -> (x/y=w288:dbl)
        n118 = Add(x=w289, y=w290) -> (x+y=w282:dbl)
        n119 = Subtract(x=w289, y=w290) -> (x-y=w291:dbl)
        n120 = Subtract(x=w288, y=w290) -> (x-y=w292:dbl)
        n121 = Add(x=w288, y=w290) -> (x+y=w295:dbl)
        n122 = Increment(x=w291) -> (x+1=w294:dbl)
        n123 = Increment(x=w292) -> (x+1=w283:dbl)
        n124 = local write "Initial Cloumn"(w294) -> ()
        n125 = local write "Final Column"(w295) -> ()
        n126 = local write "Initial Line"(w283) -> ()
        n127 = local write "Final Line"(w282) -> ()
        n128 = property on="Initial Line" class="DigNum (strict)"("DisabledEnum"=w293) -> ()  [unwired: 2 in, 2 out]
        n129 = property on="Initial Cloumn" class="DigNum (strict)"("DisabledEnum"=w293) -> ()  [unwired: 2 in, 2 out]
        n130 = property on="Final Line" class="DigNum (strict)"("DisabledEnum"=w293) -> ()  [unwired: 2 in, 2 out]
        n131 = property on="Final Column" class="DigNum (strict)"("DisabledEnum"=w293) -> ()  [unwired: 2 in, 2 out]
        n132 = flat-sequence {
          tunnel: w298 -> [w316]
          tunnel: w299 -> [w317]
          tunnel: [w317] -> w297
          tunnel: [w316] -> w296
          frame #0 {
            w310 = cluster{dbl, dbl} {0.0, 0.0}
            n133 = local read "Initial Cloumn"() -> (w309:u16)
            n134 = local read "Final Column"() -> (w307:u16)
            n135 = local read "Final Line"() -> (w308:u16)
            n136 = local read "Final Line"() -> (w306:u16)
            n137 = Bundle(cluster=w310, w309, w308) -> (w315:cluster{dbl, dbl})
            n138 = Bundle(cluster=w310, w309, w306) -> (w314:cluster{dbl, dbl})
            n139 = Bundle(cluster=w310, w307, w306) -> (w313:cluster{dbl, dbl})
            n140 = Bundle(cluster=w310, w307, w308) -> (w312:cluster{dbl, dbl})
            n141 = Bundle(cluster=w310, w309, w308) -> (w311:cluster{dbl, dbl})
            n142 = Build Array(w315, w314, w313, w312, w311) -> ()  [unwired: 1 out]
          }
        }
      }
      event "Acquisition Mode": Value Change {
        n143 = event-data() -> ("NewVal"=w319:u16)  [unwired: 1 in]
        n144 = case shown="1, Default" w319 {
          tunnel: [T6."Enabled" ("Disabled") T6."Disabled and Grayed Out" ("Disabled")] -> w318
          frame 3 {
          }
          frame 1, Default {
          }
        }
        n145 = property on="#frames" class="DigNum (strict)"("DisabledEnum"=w318) -> ()  [unwired: 2 in, 2 out]
      }
      event "Cooler": Value Change {
        n146 = event-data() -> ()  [unwired: 1 in, 1 out]
        n147 = call "Read Channel lvclass.vi"("error in (no error)"=w339, "SPARC4_GUI in"=w340) -> ("error out"=w346:errorcluster, "Channel.lvclass"=w342:refnum<class "Channel.lvclass">, "SPARC4_GUI out"=w345:refnum<class "S4GEI.lvclass">)  [unwired: 7 in]
        n148 = call-dynamic "Read Camera.lvclass.vi"("error in (no error)"=w346, "Channel in"=w342) -> ("error out"=w337:errorcluster, "Camera.lvclass"=w338:refnum<class "Camera.lvclass">, "Channel out"=w341:refnum<class "Channel.lvclass">)  [unwired: 7 in]
        n149 = Boolean To (0,1)(Boolean="Cooler") -> (0, 1=w329:i16)
        n150 = call-dynamic "Read SET parameters.vi"("error in (no error)"=w337, "Camera in"=w338) -> ("error out"=w333:errorcluster, "SET parameters"=w332:T10, "Camera out"=w334:refnum<class "Camera.lvclass">)  [unwired: 7 in]
        n151 = Bundle By Name(cluster=w332, "COOLER_POWER_STATUS"=w329) -> (w331:T10)
        n152 = call-dynamic "Write SET parameters.vi"("error in (no error)"=w333, "SET parameters"=w331, "Camera in"=w334) -> ("error out"=w335:errorcluster, "Camera out"=w336:refnum<class "Camera.lvclass">)  [unwired: 7 in]
        n153 = call-dynamic "Write Camera.lvclass.vi"("error in (no error)"=w335, "Camera.lvclass"=w336, "Channel in"=w341) -> ("error out"=w344:errorcluster, "Channel out"=w343:refnum<class "Channel.lvclass">)  [unwired: 7 in]
        n154 = call "Write Channel lvclass.vi"("error in (no error)"=w344, "Channel.lvclass"=w343, "SPARC4_GUI in"=w345) -> ("error out"=w327:errorcluster, "SPARC4_GUI out"=w328:refnum<class "S4GEI.lvclass">)  [unwired: 7 in]
        n155 = call "write request state.vi"("error in (no error)"=w327, "State"="SET_COOLER", "S4GEI in"=w328) -> ("error out"=w325:errorcluster, "S4GEI out"=w326:refnum<class "S4GEI.lvclass">)  [unwired: 7 in]
      }
      event "Temp": Value Change {
        n156 = event-data() -> ()  [unwired: 1 in, 6 out]
        n157 = call "Read Channel lvclass.vi"("error in (no error)"=w361, "SPARC4_GUI in"=w362) -> ("error out"=w368:errorcluster, "Channel.lvclass"=w364:refnum<class "Channel.lvclass">, "SPARC4_GUI out"=w367:refnum<class "S4GEI.lvclass">)  [unwired: 7 in]
        n158 = call-dynamic "Read Camera.lvclass.vi"("error in (no error)"=w368, "Channel in"=w364) -> ("error out"=w359:errorcluster, "Camera.lvclass"=w360:refnum<class "Camera.lvclass">, "Channel out"=w363:refnum<class "Channel.lvclass">)  [unwired: 7 in]
        n159 = call-dynamic "Read SET parameters.vi"("error in (no error)"=w359, "Camera in"=w360) -> ("error out"=w355:errorcluster, "SET parameters"=w354:T10, "Camera out"=w356:refnum<class "Camera.lvclass">)  [unwired: 7 in]
        n160 = Bundle By Name(cluster=w354, "TEMP"="Temp") -> (w353:T10)
        n161 = call-dynamic "Write SET parameters.vi"("error in (no error)"=w355, "SET parameters"=w353, "Camera in"=w356) -> ("error out"=w357:errorcluster, "Camera out"=w358:refnum<class "Camera.lvclass">)  [unwired: 7 in]
        n162 = call-dynamic "Write Camera.lvclass.vi"("error in (no error)"=w357, "Camera.lvclass"=w358, "Channel in"=w363) -> ("error out"=w366:errorcluster, "Channel out"=w365:refnum<class "Channel.lvclass">)  [unwired: 7 in]
        n163 = call "Write Channel lvclass.vi"("error in (no error)"=w366, "Channel.lvclass"=w365, "SPARC4_GUI in"=w367) -> ("error out"=w351:errorcluster, "SPARC4_GUI out"=w352:refnum<class "S4GEI.lvclass">)  [unwired: 7 in]
        n164 = call "write request state.vi"("error in (no error)"=w351, "State"="SET_TEMP", "S4GEI in"=w352) -> ("error out"=w349:errorcluster, "S4GEI out"=w350:refnum<class "S4GEI.lvclass">)  [unwired: 7 in]
      }
    }
    n165 = Unbundle By Name(w13) -> ("status"=w18:bool)
    n166 = Or(x=w18, y="Stop Application") -> (x .or. y?=w19:bool)
  }
  n167 = Unbundle By Name(w9) -> ("source"=→"Error Message":string)
  n168 = call <vilib>:"Clear Errors.vi"("error in (no error)"=w9) -> ("error out"=w8:errorcluster)  [unwired: 5 in, 1 out]
  n169 = call "End.vi"("error in (no error)"=w8, "SPARC4_GUI in"=w11) -> ("SPARC4_GUI out"=w12:refnum<class "S4GEI.lvclass">)  [unwired: 8 in, 1 out]
  n170 = flat-sequence {
    tunnel: w12 -> [_]
    frame #0 {
      w371 = 1
      w374 = ""
      w375 = FALSE ("analyser status")
      (unwired) 0.0 ("Scale.Range:Minimum")
      (unwired) 1.0 ("Scale.Range:Maximum")
      (unwired) 1.0 ("Scale.Range:Maximum")
      (unwired) T6."Disabled and Grayed Out" ("Disabled")
      w380 = u16 0 items=["Internal", "External", "N/A", "N/A", "N/A", "N/A", "External Start", "External Exposure (Bulb)", "N/A", "External FVB EM", "Software", "N/A", "External Charge Shifting"] ("Trigger Mode")
      w381 = u16 4 items=["Full Vertical Binning", "Multi-Track", "Random-Track", "Single-Track", "Image"] ("Read Mode")
      w382 = u16 3 items=["Reserved", "Single Scan", "Accumulate", "Kinetic", "Fast Kinetic", "Run till abort", "Reserved", "Reserved", "Reserved", "Time Delayed Integration"] ("Acquisition Mode")
      w387 = u16 0 items=["TTL Low", "TTL High"] ("Shutter TTL")
      w388 = u8 0 items=["  1 MHz", "0.1 MHz"] ("Readout Rate")
      w390 = u8 2 items=["Fully Auto", "OPEN", "CLOSED"] ("Shutter Mode")
      w373 = "" ("Command:")
      w392 = u16 1024 ("Final Line")
      w391 = u16 1 ("Initial Cloumn")
      w395 = u8 0 items=["Gain 1", "Gain 2"] ("Pre-amp gain")
      n171 = local write "#frames"(w371) -> ()
      n172 = local write "#cycles"(w371) -> ()
      n173 = property on="Cycles done" class="Slide (strict)"("Scale.Maximum"=1.0 ("Scale.Range:Maximum")) -> ()  [unwired: 2 in, 2 out]
      n174 = property on="Frames done" class="Slide (strict)"("Scale.Maximum"=1.0 ("Scale.Range:Maximum")) -> ()  [unwired: 2 in, 2 out]
      n175 = local write "CCD status"(T13 {"Cycles done"=1, "Frames done"=1, "CCD Status"="", "Exposing"=FALSE, "Last image"="", "temp"=0, "serial n"=0, "texp"=0.0, "used disk"=0, "Power"=FALSE, "ACS mode"=FALSE} ("CCD status 2")) -> ()
      n176 = property on="temp" class="DigNum (strict)"("NumText.BGColor"=u32 12369084) -> ()  [unwired: 2 in, 2 out]
      n177 = local write "Command:"(w373) -> ()
      n178 = local write "observer"(w373) -> ()
      n179 = local write "projid"(w373) -> ()
      n180 = local write "file name suffix"(w374) -> ()
      n181 = local write "object name"(w374) -> ()
      n182 = local write "comment"(w374) -> ()
      n183 = property on="acs mode" class="Bool (strict)"("Colors [4]"=cluster{u32, u32}[] [{1985280, 1985280}, {1985280, 1985280}, {6618880, 6618880}]) -> ()  [unwired: 2 in, 2 out]
      n184 = local write "preset modes"(T14 {"object"=FALSE, "test"=FALSE, "zero"=FALSE, "dark"=FALSE, "sflat"=FALSE, "dflat"=FALSE, "focus"=FALSE, "led object"=FALSE, "led test"=FALSE, "led zero"=FALSE, "led dark"=FALSE, "led sflat"=FALSE, "led dflat"=FALSE, "led foc"=FALSE} ("preset modes")) -> ()
      n185 = local write "start exp"(w375) -> ()
      n186 = local write "Stop Acquisition"(w375) -> ()
      n187 = local write "Abort Acquisition"(w375) -> ()
      n188 = local write "Pause acquisition"(w375) -> ()
      n189 = local write "Shutter TTL"(w387) -> ()
      n190 = local write "Shutter Time"(u16 50 ("Shutter Time")) -> ()
      n191 = local write "Vertical Shift Speed"(u16 3 ("Vertical Shift Speed")) -> ()
      n192 = local write "AD Channel"(u16 0 ("AD Channel")) -> ()
      n193 = local write "Vertical Clock Voltagem"(u16 0 ("Vertical Clock Voltagem")) -> ()
      n194 = local write "Acquisition Mode"(w382) -> ()
      n195 = local write "Read Mode"(w381) -> ()
      n196 = local write "Trigger Mode"(w380) -> ()
      n197 = property on="Readout Rate" class="Ring (strict)"("Strings []"=string[] ["1 MHz", "0.1 MHz"]) -> ()  [unwired: 2 in, 2 out]
      n198 = local write "Shutter Mode"(w390) -> ()
      n199 = local write "Readout Rate"(w388) -> ()
      n200 = local write "Pre-amp gain"(w395) -> ()
      n201 = local write "Sub Image"(T3."1024 x 1024" ("Sub Image")) -> ()
      n202 = local write "Initial Line"(u16 1 ("Initial Line")) -> ()
      n203 = local write "Final Line"(w392) -> ()
      n204 = local write "Final Column"(w392) -> ()
      n205 = local write "Initial Cloumn"(w391) -> ()
      n206 = local write "Binning"(w391) -> ()
      n207 = property on="#frames" class="DigNum (strict)"("DisabledEnum"=T6."Enabled" ("Disabled")) -> ()  [unwired: 2 in, 2 out]
    }
  }
